vi "ControlStyleReference.vi"() -> ()   [LabVIEW 2013]
panel:
  out "Style ID 8":u32
  in  "Cluster":cluster{"Numeric":dbl, "String":string}
  out "Style ID 7":u32
  in  "refNum":refnum<vi>
  in  "Array 3":string[](array[string])
  out "Style ID 6":u32
  in  "Array 2":bool[](array[boolean])
  out "Style ID 5":u32
  in  "Array":dbl[](array[numeric])
  in  "String":string
  in  "Boolean":bool
  out "Style ID 4":u32
  out "Style ID 3":u32
  out "Style ID 2":u32
  out "Style ID":u32
  in  "Numeric":dbl
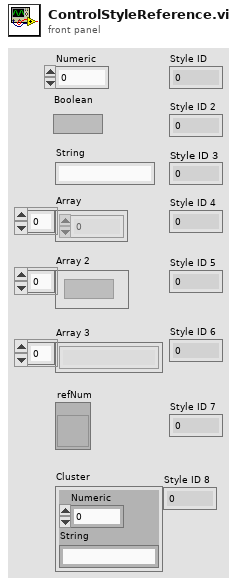
[diagram p1: front panel]
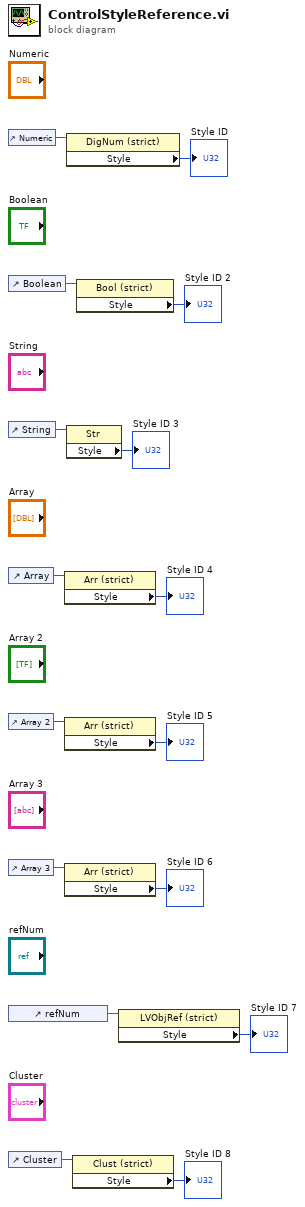
[diagram p0: block diagram]
diagram:
  n1 = control-ref of="Numeric"() -> (w16:refnum<vi>)
  n2 = control-ref of="Boolean"() -> (w11:refnum<vi>)
  n3 = control-ref of="String"() -> (w10:refnum<vi>)
  n4 = control-ref of="Array"() -> (w9:refnum<vi>)
  n5 = control-ref of="Array 2"() -> (w7:refnum<vi>)
  n6 = control-ref of="Array 3"() -> (w5:refnum<vi>)
  n7 = control-ref of="refNum"() -> (w4:refnum<vi>)
  n8 = control-ref of="Cluster"() -> (w1:refnum<vi>)
  n9 = property class="Arr (strict)"(reference=w9) -> ("Style"=→"Style ID 4":u32)  [unwired: 1 in, 2 out]
  n10 = property class="Arr (strict)"(reference=w7) -> ("Style"=→"Style ID 5":u32)  [unwired: 1 in, 2 out]
  n11 = property class="Arr (strict)"(reference=w5) -> ("Style"=→"Style ID 6":u32)  [unwired: 1 in, 2 out]
  n12 = property class="DigNum (strict)"(reference=w16) -> ("Style"=→"Style ID":u32)  [unwired: 1 in, 2 out]
  n13 = property class="Str"(reference=w10) -> ("Style"=→"Style ID 3":u32)  [unwired: 1 in, 2 out]
  n14 = property class="Clust (strict)"(reference=w1) -> ("Style"=→"Style ID 8":u32)  [unwired: 1 in, 2 out]
  n15 = property class="Bool (strict)"(reference=w11) -> ("Style"=→"Style ID 2":u32)  [unwired: 1 in, 2 out]
  n16 = property class="LVObjRef (strict)"(reference=w4) -> ("Style"=→"Style ID 7":u32)  [unwired: 1 in, 2 out]
